vi "saveToFile.vi"(9 "SigJSONbuffer":string, 10 "dimensions":i64[](array[numeric]), 11 "String":string) -> (0 "error out":errorcluster, 1 "resulting string":string)   [LabVIEW 2014]
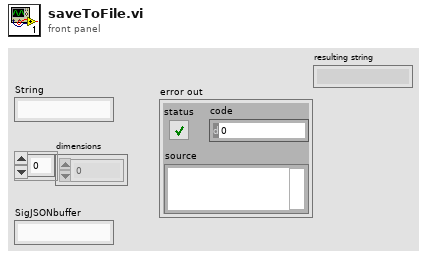
[diagram p1: front panel]
types:
  T1 = enum16{"open", "replace", "create", "open or create", "replace or create", "replace or create with confirmation"}
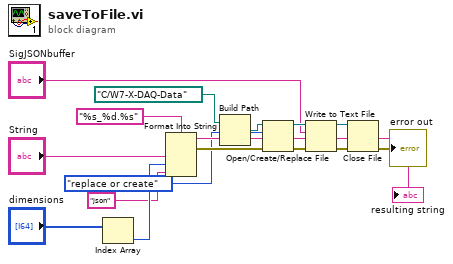
[diagram p0: block diagram]
diagram:
  n1 = Index Array(array="dimensions") -> (element=w14:i64)  [unwired: 1 in]
  n2 = Format Into String(format string="%s_%d.%s", "String", w14, "json" ("input 3")) -> (resulting string=w16:string, error out=w15:errorcluster)  [unwired: 2 in]
  "resulting string" <- w16
  n3 = Build Path(base path=path "C:/W7-X-DAQ-Data", name or relative path=w16) -> (appended path=w11:path)
  n4 = Open/Create/Replace File(file path (use dialog)=w11, error in=w15, operation (0:open)=T1."replace or create") -> (refnum out=w9:refnum<file>, error out=w10:errorcluster)  [unwired: 3 in, 1 out]
  n5 = Write to Text File(file (use dialog)=w9, text="SigJSONbuffer", error in=w10) -> (refnum out=w8:refnum<file>, error out=w6:errorcluster)  [unwired: 1 in, 1 out]
  n6 = Close File(refnum=w8, error in=w6) -> (error out=→"error out":errorcluster)  [unwired: 1 out]
